vi "Strip_string.vi"(0 "Oscilloscope Setting Information Normal mode":string) -> (1 "Settings":T1, 2 "Autoscale?":i8, 3 "Remaining string":string)   [LabVIEW 2011]
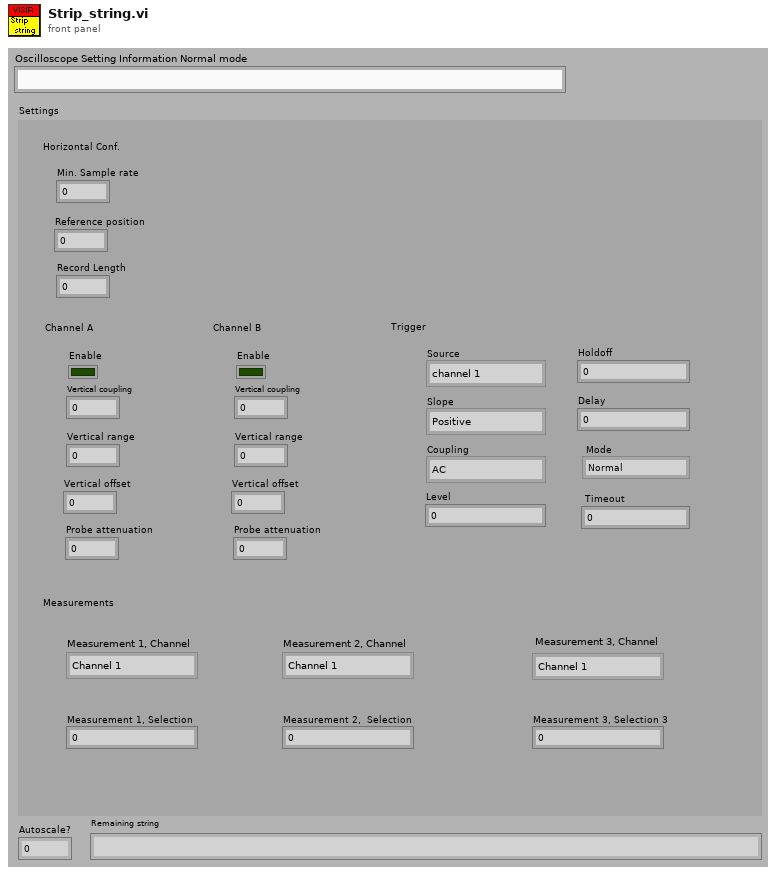
[diagram p1: front panel]
types:
  T1 = cluster{"Horizontal Conf.":cluster{"Min. Sample rate":dbl, "Reference position":dbl, "Record Length":i16}, "Channel A":cluster{"Enable":bool, "Vertical coupling":i32, "Vertical range":dbl, "Vertical offset":dbl, "Probe attenuation":dbl}, "Channel B":cluster{"Enable":bool, "Vertical coupling":i32, "Vertical range":dbl, "Vertical offset":dbl, "Probe attenuation":dbl}, "Trigger":cluster{"Source":enum8{"channel 1", "channel 2", "Imediate", "External trigger"}, "Slope":enum8{"Positive", "Negative"}, "Coupling":enum8{"AC", "DC"}, "Level":dbl, "Holdoff":dbl, "Delay":dbl, " Timeout":dbl, " Mode":enum8{"Normal", "Auto", "Auto Level", ""}}, "Measurements":cluster{"Measurement 1, Channel":enum8{"Channel 1", "Channel 2", "Channel 3", "Channel 4"}, "Measurement 1, Selection":u16, "Measurement 2, Channel":enum8{"Channel 1", "Channel 2", "Channel 3", "Channel 4"}, "Measurement 2,  Selection":u16, "Measurement 3, Channel":enum8{"Channel 1", "Channel 2", "Channel 3", "Channel 4"}, "Measurement 3, Selection 3":u16}}
  T2 = cluster{cluster{dbl, dbl, dbl}, cluster{bool, dbl, dbl, dbl, dbl}, cluster{bool, dbl, dbl, dbl, dbl}, cluster{dbl, dbl, dbl, dbl, dbl, dbl, dbl, dbl}, cluster{dbl, dbl, dbl, dbl, dbl, dbl}}
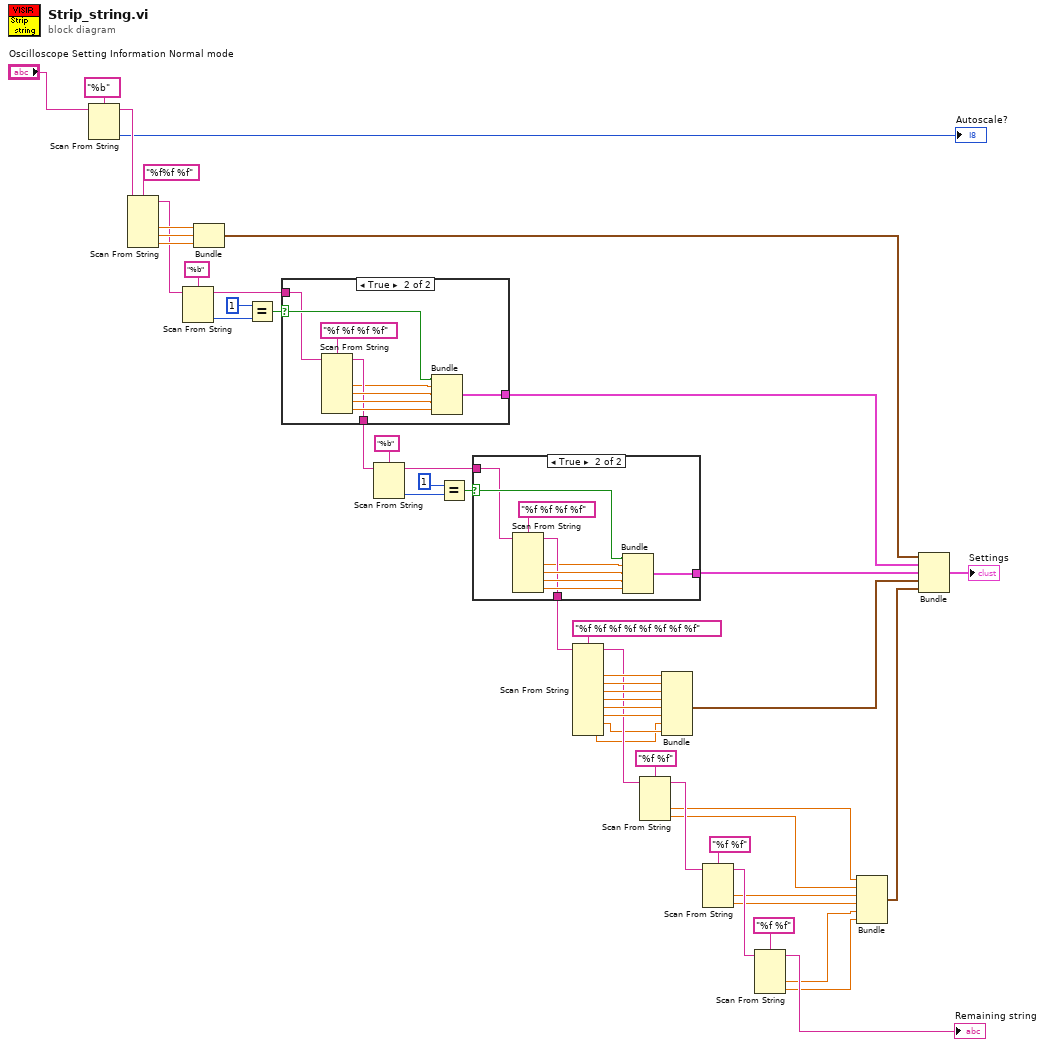
[diagram p0: block diagram]
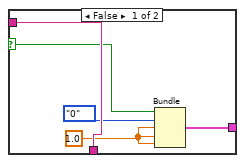
[diagram p2: hidden frame]
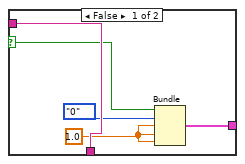
[diagram p3: hidden frame]
diagram:
  n1 = Scan From String(format string="%b", input string="Oscilloscope Setting Information Normal mode") -> (remaining string=w14:string, output 1=→"Autoscale?":i8)  [unwired: 3 in, 2 out]
  n2 = Scan From String(format string="%f%f %f", input string=w14) -> (remaining string=w36:string, output 1=w48:dbl, output 2=w47:dbl, output 3=w46:dbl)  [unwired: 5 in, 2 out]
  n3 = Scan From String(format string="%b", input string=w36) -> (remaining string=w32:string, output 1=w31:i32)  [unwired: 3 in, 2 out]
  n4 = Bundle(w48, w47, w46) -> (w22:cluster{dbl, dbl, dbl})  [unwired: 1 in]
  n5 = Equal?(x=1, y=w31) -> (x = y?=w33:bool)
  n6 = case shown="True" w33 {
    selector: w33 -> [w52 w57]
    tunnel: w32 -> [w54 w55]
    tunnel: [w53 w59] -> w21
    tunnel: [w54 w58] -> w25
    frame False {
      w51 = 1.0
      n7 = Bundle(w52, enum16{"0"}."0", w51, w51, w51) -> (w53:cluster{bool, enum16{"0"}, dbl, dbl, dbl})  [unwired: 1 in]
    }
    frame True {
      n8 = Scan From String(format string="%f %f %f %f", input string=w55) -> (remaining string=w58:string, output 1=w56:dbl, output 2=w62:dbl, output 3=w61:dbl, output 4=w60:dbl)  [unwired: 6 in, 2 out]
      n9 = Bundle(w57, w56, w62, w61, w60) -> (w59:cluster{bool, dbl, dbl, dbl, dbl})  [unwired: 1 in]
    }
  }
  n10 = Scan From String(format string="%b", input string=w25) -> (remaining string=w27:string, output 1=w26:i32)  [unwired: 3 in, 2 out]
  n11 = Equal?(x=1, y=w26) -> (x = y?=w28:bool)
  n12 = case shown="True" w28 {
    selector: w28 -> [w66 w71]
    tunnel: w27 -> [w68 w69]
    tunnel: [w67 w73] -> w20
    tunnel: [w68 w72] -> w24
    frame False {
      w65 = 1.0
      n13 = Bundle(w66, enum16{"0"}."0", w65, w65, w65) -> (w67:cluster{bool, enum16{"0"}, dbl, dbl, dbl})  [unwired: 1 in]
    }
    frame True {
      n14 = Scan From String(format string="%f %f %f %f", input string=w69) -> (remaining string=w72:string, output 1=w70:dbl, output 2=w76:dbl, output 3=w75:dbl, output 4=w74:dbl)  [unwired: 6 in, 2 out]
      n15 = Bundle(w71, w70, w76, w75, w74) -> (w73:cluster{bool, dbl, dbl, dbl, dbl})  [unwired: 1 in]
    }
  }
  n16 = Scan From String(format string="%f %f %f %f %f %f %f %f", input string=w24) -> (remaining string=w39:string, output 1=w45:dbl, output 2=w43:dbl, output 3=w44:dbl, output 4=w41:dbl, output 5=w42:dbl, output 6=w40:dbl, output 7=w18:dbl, output 8=w17:dbl)  [unwired: 10 in, 2 out]
  n17 = Scan From String(format string="%f %f", input string=w39) -> (remaining string=w38:string, output 1=w8:dbl, output 2=w7:dbl)  [unwired: 4 in, 2 out]
  n18 = Bundle(w45, w43, w44, w41, w42, w40, w17, w18) -> (w19:cluster{dbl, dbl, dbl, dbl, dbl, dbl, dbl, dbl})  [unwired: 1 in]
  n19 = Scan From String(format string="%f %f", input string=w38) -> (remaining string=w37:string, output 1=w6:dbl, output 2=w5:dbl)  [unwired: 4 in, 2 out]
  n20 = Scan From String(format string="%f %f", input string=w37) -> (remaining string=→"Remaining string":string, output 1=w4:dbl, output 2=w3:dbl)  [unwired: 4 in, 2 out]
  n21 = Bundle(w8, w7, w6, w5, w4, w3) -> (w1:cluster{dbl, dbl, dbl, dbl, dbl, dbl})  [unwired: 1 in]
  n22 = Bundle(w22, w21, w20, w19, w1) -> (→"Settings":T2)  [unwired: 1 in]
